vi "Unregister Sessions.vi"(8 "error in":errorcluster, 11 "session reservation in":refnum<class "Session Reservation.lvclass">) -> (0 "error out":errorcluster, 3 "session reservation out":refnum<class "Session Reservation.lvclass">)   [LabVIEW 2020, in "MeasurementLink Session Management.lvlib" / "Session Reservation.lvclass"]
doc: "Unregisters sessions with the session management service."
uses:
  Session Reservation.lvclass
  Session Reservation.lvclass/Session Reservation.ctl
  MeasurementLink Session Management Client/RPC Messages/ni_measurementlink_sessionmanagement_v1_UnregisterSessionsRequest.ctl
  MeasurementLink Session Management Client/RPC Messages/ni_measurementlink_sessionmanagement_v1_SessionInformation.ctl
  MeasurementLink Session Management Client/RPC Messages/nidevice_grpc_Session.ctl
  MeasurementLink Session Management Client/RPC Messages/ni_measurementlink_sessionmanagement_v1_ChannelMapping.ctl
  MeasurementLink Measurement Server/Helpers/Error Strings Global Internal.vi
  <vilib>/Utility/error.llb/Error Cluster From Error Code.vi
  MeasurementLink Session Management Client/MeasurementLink Session Management Client.lvlib
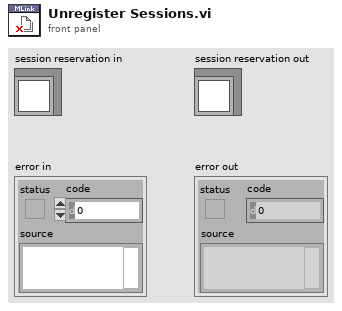
[diagram p1: front panel]
types:
  T1 = typedef "MeasurementLink Session Management Client.lvlib/ni_measurementlink_sessionmanagement_v1_UnregisterSessionsRequest.ctl" = cluster{"sessions":T2[]}
  T2 = typedef "MeasurementLink Session Management Client.lvlib/ni_measurementlink_sessionmanagement_v1_SessionInformation.ctl" = cluster{"session":T3, "resource_name":string, "channel_list":string, "instrument_type_id":string, "session_exists":bool, "channel_mappings":T4[]}
  T3 = typedef "MeasurementLink Session Management Client.lvlib/nidevice_grpc_Session.ctl" = cluster{"name":string}
  T4 = typedef "MeasurementLink Session Management Client.lvlib/ni_measurementlink_sessionmanagement_v1_ChannelMapping.ctl" = cluster{"pin_or_relay_name":string, "site":i32, "channel":string}
  T5 = typedef "MeasurementLink Session Management.lvlib/Session Reservation.lvclass/Data.ctl" = cluster{"session and driver infos":T6[], "pin or relay names":string[], "connection map":refnum<class "Connection Map.lvclass">, "pin map context":T8, "reservation observer":refnum<class "IReservationObserver.lvclass">, "dvr valid":bool}
  T6 = typedef "MeasurementLink Session Management.lvlib/Session Reservation.lvclass/Session and Driver Info.ctl" = cluster{"session info":T2, "session":variant, "session factory":refnum<class "ISession Factory.lvclass">, "initialize and close session behavior":T7}
  T7 = typedef "MeasurementLink Instrument.lvlib/ISession Factory.lvclass/Initialize and Close Session Behavior.ctl" = enum16{"Initialize and Close", "Attach and Detach", "Initialize and Detach", "Attach and Close"}
  T8 = typedef "MeasurementLink Session Management Client.lvlib/ni_measurementlink_PinMapContext.ctl" = cluster{"pin_map_id":string, "sites":i32[]}
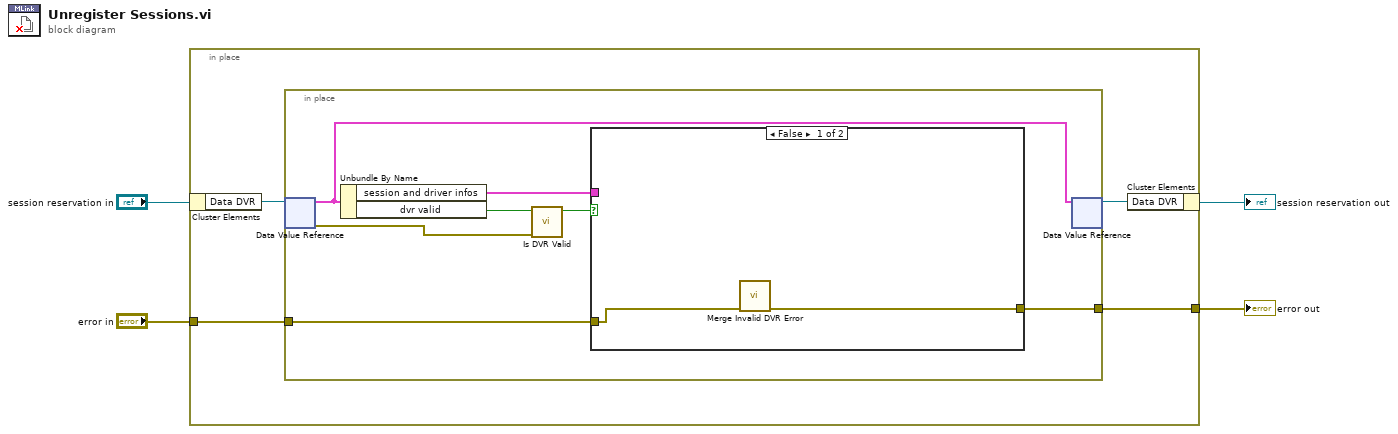
[diagram p0: block diagram]
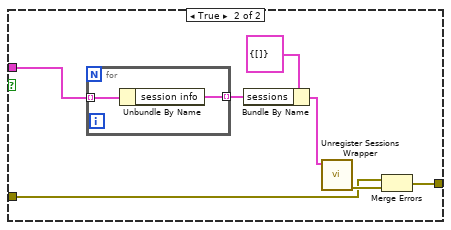
[diagram p2: hidden frame]
diagram:
  n1 = in-place {
    in-place-border: "error in" -> [w8]
    in-place-border: [w7] -> w3
    n2 = in-place-cluster #1("session reservation in") -> ("Data DVR"=w6:refnum<data-value>)
    n3 = in-place {
      in-place-border: w8 -> [w13]
      in-place-border: [w12] -> w7
      n4 = in-place-dvr #2(w6) -> (w9:T5, w14:errorcluster)
      n5 = Unbundle By Name(w9) -> ("session and driver infos"=w10:T6[], "dvr valid"=w11:bool)
      n6 = call "Is DVR Valid.vi"("dvr error in"=w14, "dvr valid"=w11) -> ("dvr valid"=w15:bool)  [unwired: 9 in]
      n7 = case shown="False" w15 {
        tunnel: w13 -> [w17 w20]
        tunnel: [w16 w19] -> w12
        tunnel: w10 -> [_ w18]
        frame False {
          n8 = call "Merge Invalid DVR Error.vi"("error in (no error)"=w17) -> ("error out"=w16:errorcluster)  [unwired: 10 in]
        }
        frame True {
          n9 = for {
            tunnel: w18 -> [w26] mode=indexing
            tunnel: [w25] -> w23 mode=indexing
            n10 = Unbundle By Name(w26) -> ("session info"=w25:T2)
          }
          n11 = Bundle By Name(cluster=T1 {"sessions"=[]} ("Request Data"), "sessions"=w23) -> (w22:T1)
          n12 = call "Unregister Sessions Wrapper.vi"("request data"=w22) -> ("error out"=w21:errorcluster)  [unwired: 9 in, 1 out]
          n13 = Merge Errors(w20, w21) -> (w19:errorcluster)
        }
      }
      n14 = in-place-dvr #2(w9) -> (w5:refnum<data-value>)  [unwired: 1 out]
    }
    n15 = in-place-cluster #1("Data DVR"=w5) -> (→"session reservation out":refnum<class "Session Reservation.lvclass">)
  }
  "error out" <- w3
